vi "sendStopServerNotifier.vi"(8 "error in (no error)":errorcluster, 11 "TcpServerTel in":refnum<class "TcpServerTel.lvclass">) -> (0 "error out":errorcluster, 3 "TcpServerTel out":refnum<class "TcpServerTel.lvclass">)   [LabVIEW 2018, in "TcpServerTel.lvclass"]
doc: "Send the stopServerTel notifier to stop the runServer.vi."
uses:
  TcpServerTel.lvclass
  home/pcortes/Documents/github/ts_labview_tcp_json/src/TcpServerBase/TcpServerBase.lvclass
  TcpServerBase/TcpServerBase.lvclass
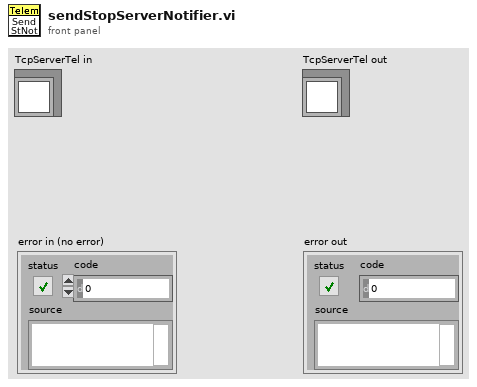
[diagram p1: front panel]
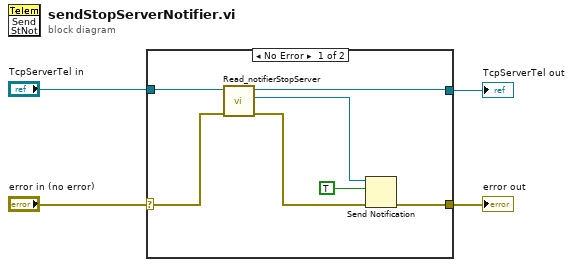
[diagram p0: block diagram]
diagram:
  n1 = case shown="No Error" "error in (no error)" {
    selector: "error in (no error)" -> [w8 w13]
    tunnel: "TcpServerTel in" -> [w9 w12]
    tunnel: [w11 w13] -> w3
    tunnel: [w7 w12] -> w1
    frame No Error {
      n2 = call "Read_notifierStopServer.vi"("error in (no error)"=w8, "TcpServerBase in"=w9) -> ("error out"=w6:errorcluster, "stopServerNotifier"=w5:refnum<notifier>, "TcpServerBase out"=w7:refnum<class "TcpServerTel.lvclass">)  [unwired: 7 in]
      n3 = Send Notification(notification=TRUE, notifier=w5, error in (no error)=w6) -> (error out=w11:errorcluster)  [unwired: 1 out]
    }
    frame Error {
    }
  }
  "error out" <- w3
  "TcpServerTel out" <- w1
